vi "SSC Digital Read Static.vi"(0 "Digital SSC in":T2[](array[typedef]), 11 "error in":errorcluster) -> (4 "Digital SSC out":T2[](array[typedef]), 6 "Per-Instrument Data":T1[][](array[typedef]) items=["0"=0, "1"=1, "L"=3, "H"=4, "X"=5, "M"=6, "V"=7, "D"=8, "E"=9, "Not A Pin State"=254], 15 "error out":errorcluster)   [LabVIEW 2019]
doc: "Reads the current state of comparators for the specified pin(s) and pin group(s). If there are uncommitted changes to levels or the termination mode, this VI commits the changes to the pins."
uses:
  SSC Digital.ctl
  <instrlib>/niDigital/niDigital.llb/niDigital Pin State.ctl
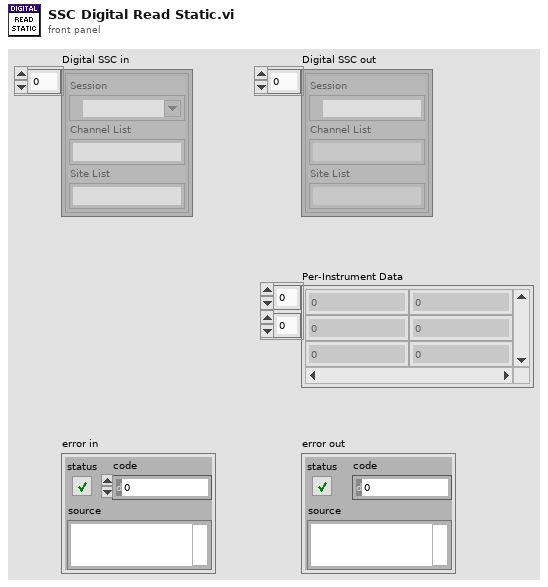
[diagram p1: front panel]
types:
  T1 = typedef "niDigital Pin State.ctl" = u8
  T2 = typedef "SSC Digital.ctl" = cluster{"Session":refnum<k15>, "Channel List":string, "Site List":string}
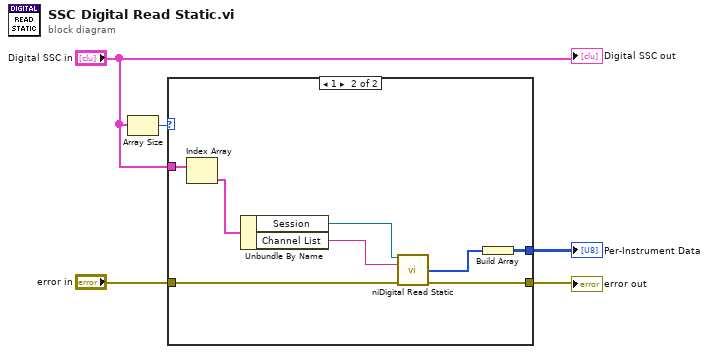
[diagram p0: block diagram]
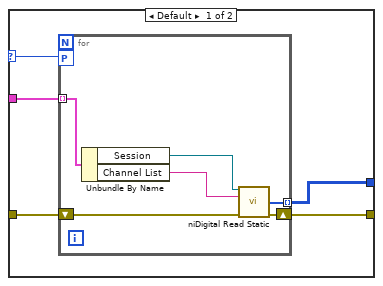
[diagram p2: hidden frame]
diagram:
  n1 = Array Size(array="Digital SSC in") -> (size(s)=w2:i32)
  n2 = case shown="1" w2 {
    selector: w2 -> [w7 _]
    tunnel: "error in" -> [w10 w24]
    tunnel: [w9 w23] -> w4
    tunnel: [w8 w17] -> w3
    tunnel: "Digital SSC in" -> [w6 w21]
    frame Default {
      n3 = for {
        workers-P: w7 -> [_]
        tunnel: w6 -> [w14] mode=indexing
        shift-right: [w15] -> w9
        shift-left: w10 -> [w16]
        tunnel: [w11] -> w8 mode=indexing
        n4 = Unbundle By Name(w14) -> ("Session"=w12:refnum<k15>, "Channel List"=w13:string)
        n5 = call <instrlib>:"niDigital Read Static.vi"("instrument handle"=w12, "channel list"=w13, "error in"=w16) -> ("data"=w11:T1[], "error out"=w15:errorcluster)  [unwired: 10 in, 1 out]
      }
    }
    frame 1 {
      n6 = Index Array(array=w21) -> (element=w18:T2)  [unwired: 1 in]
      n7 = Unbundle By Name(w18) -> ("Session"=w19:refnum<k15>, "Channel List"=w20:string)
      n8 = call <instrlib>:"niDigital Read Static.vi"("instrument handle"=w19, "channel list"=w20, "error in"=w24) -> ("data"=w22:T1[], "error out"=w23:errorcluster)  [unwired: 10 in, 1 out]
      n9 = Build Array(w22) -> (w17:T1[][])
    }
  }
  "error out" <- w4
  "Per-Instrument Data" <- w3
  "Digital SSC out" <- "Digital SSC in"
